vi "0-35_v2 (SubVI).vi"(1 "String":string) -> (0 "color":u32[](array[colorbox]))   [LabVIEW 2024]
panel:
  in  "Numeric":i32
  out "2":u32[](array[numeric])
  in  "Array in":refnum<vi>
  out "1 o":u32[](array[numeric])
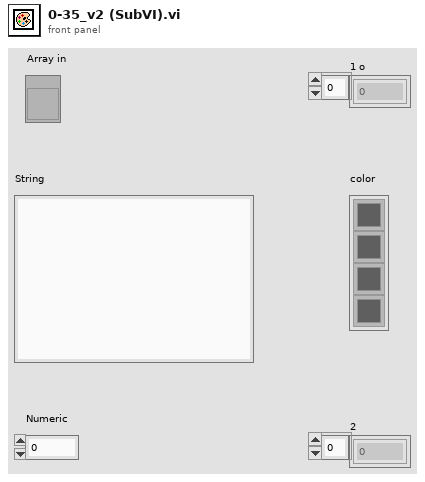
[diagram p1: front panel]
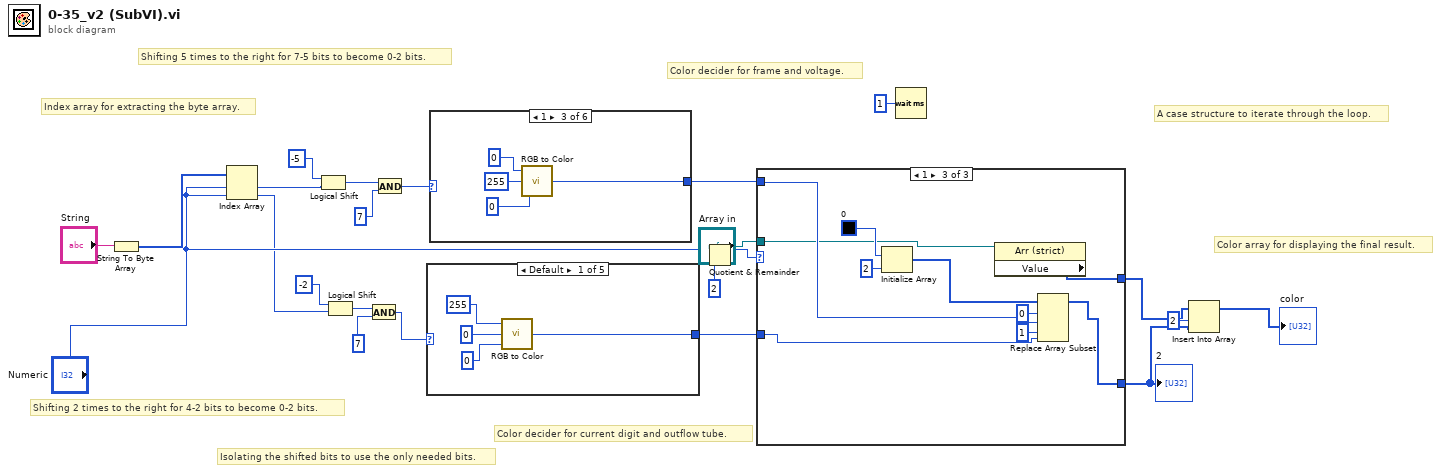
[diagram p0: block diagram]
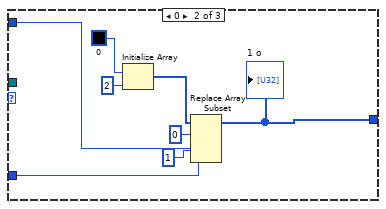
[diagram p3: hidden frame]
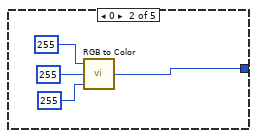
[diagram p4: hidden frame]
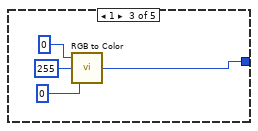
[diagram p5: hidden frame]
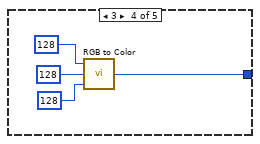
[diagram p6: hidden frame]
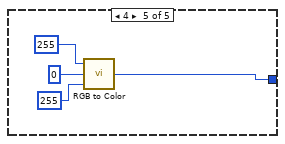
[diagram p7: hidden frame]
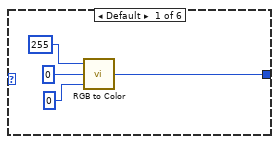
[diagram p8: hidden frame]
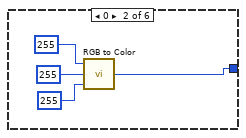
[diagram p9: hidden frame]
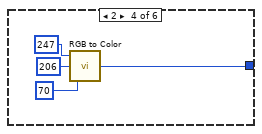
[diagram p10: hidden frame]
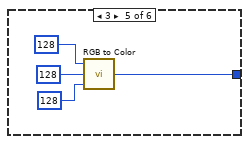
[diagram p11: hidden frame]
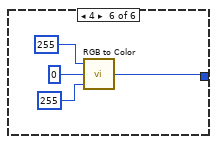
[diagram p12: hidden frame]
diagram:
  # "A case structure to iterate through the loop."
  # "Color array for displaying the final result."
  # "Index array for extracting the byte array."
  # "Color decider for current digit and outflow tube."
  # "Color decider for frame and voltage."
  # "Isolating the shifted bits to use the only needed bits."
  # "Shifting 2 times to the right for 4-2 bits to become 0-2 bits."
  # "Shifting 5 times to the right for 7-5 bits to become 0-2 bits."
  n1 = String To Byte Array(string="String") -> (unsigned byte array=w20:u8[])
  n2 = Index Array(array=w20, index #1="Numeric", index #2="Numeric") -> (element #1=w7:u8, element #2=w9:u8)
  n3 = Logical Shift(y=i16 -5, x=w7) -> (x << y=w11:u8)
  n4 = Logical Shift(y=i16 -2, x=w9) -> (x << y=w5:u8)
  n5 = And(x=w5, y=u8 7) -> (x .and. y?=w8:u8)
  n6 = And(x=w11, y=u8 7) -> (x .and. y?=w10:u8)
  n7 = case shown="Default" w8 {
    tunnel: [w24 w28 w32 w36 w41] -> w13
    frame Default {
      n8 = call <vilib>:"RGB to Color.vi"("B"=u8 0, "G"=u8 0, "R"=u8 255) -> ("Color"=w24:u32)
    }
    frame 0 {
      n9 = call <vilib>:"RGB to Color.vi"("B"=u8 255, "G"=u8 255, "R"=u8 255) -> ("Color"=w28:u32)
    }
    frame 1 {
      n10 = call <vilib>:"RGB to Color.vi"("B"=u8 0, "G"=u8 255, "R"=u8 0) -> ("Color"=w32:u32)
    }
    frame 3 {
      n11 = call <vilib>:"RGB to Color.vi"("B"=u8 128, "G"=u8 128, "R"=u8 128) -> ("Color"=w36:u32)
    }
    frame 4 {
      n12 = call <vilib>:"RGB to Color.vi"("B"=u8 255, "G"=u8 0, "R"=u8 255) -> ("Color"=w41:u32)
    }
  }
  n13 = case shown="1" w10 {
    tunnel: [w44 w48 w52 w56 w60 w64] -> w12
    frame Default {
      n14 = call <vilib>:"RGB to Color.vi"("B"=u8 0, "G"=u8 0, "R"=u8 255) -> ("Color"=w44:u32)
    }
    frame 0 {
      n15 = call <vilib>:"RGB to Color.vi"("B"=u8 255, "G"=u8 255, "R"=u8 255) -> ("Color"=w48:u32)
    }
    frame 1 {
      n16 = call <vilib>:"RGB to Color.vi"("B"=u8 0, "G"=u8 255, "R"=u8 0) -> ("Color"=w52:u32)
    }
    frame 2 {
      n17 = call <vilib>:"RGB to Color.vi"("B"=u8 70, "G"=u8 206, "R"=u8 247) -> ("Color"=w56:u32)
    }
    frame 3 {
      n18 = call <vilib>:"RGB to Color.vi"("B"=u8 128, "G"=u8 128, "R"=u8 128) -> ("Color"=w60:u32)
    }
    frame 4 {
      n19 = call <vilib>:"RGB to Color.vi"("B"=u8 255, "G"=u8 0, "R"=u8 255) -> ("Color"=w64:u32)
    }
  }
  n20 = Quotient & Remainder(x="Numeric", y=2) -> (x-y*floor(x/y)=w21:i32)  [unwired: 1 out]
  n21 = case shown="1" w21 {
    tunnel: [_ w68 w77] -> w15
    tunnel: w12 -> [_ w72 w82]
    tunnel: w13 -> [_ w71 w81]
    tunnel: [_ _ w80] -> w16
    tunnel: "Array in" -> [_ _ w76]
    frame Default {
    }
    frame 0 {
      n22 = Initialize Array(u32 0, 2 ("dimension size")) -> (w73:u32[])
      n23 = Replace Array Subset(array=w73, new element #1=w72, index #1=0 ("index"), new element #2=w71, index #2=1 ("index")) -> (w68:u32[])
      "1 o" <- w68
    }
    frame 1 {
      n24 = Initialize Array(u32 0, 2 ("dimension size")) -> (w84:u32[])
      n25 = property class="Arr (strict)"(reference=w76) -> ("Value"=w77:u32[])  [unwired: 1 in, 2 out]
      n26 = Replace Array Subset(array=w84, new element #1=w82, index #1=0 ("index"), new element #2=w81, index #2=1 ("index")) -> (w80:u32[])
    }
  }
  "2" <- w16
  n27 = Wait (ms)(milliseconds to wait=u32 1) -> ()  [unwired: 1 out]
  n28 = Insert Into Array(array=w15, index=2, new element=w16) -> (→"color":u32[])
